vi "Create Tones.vi"(0 "ToneCloud in":refnum<class "Tone Cloud.lvclass">, 9 "Fs (Hz)":dbl, 11 "error in (no error)":errorcluster) -> (4 "ToneCloud out":refnum<class "Tone Cloud.lvclass">, 15 "error out":errorcluster)   [LabVIEW 2020, in "Tone Cloud.lvclass"]
uses:
  Tone Cloud.lvclass
  Tone Cloud.lvclass/Tone Cloud.ctl
  <vilib>/Analysis/NI_AALBase.lvlib
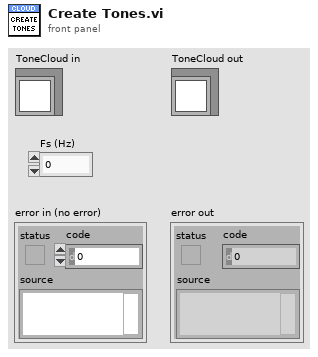
[diagram p1: front panel]
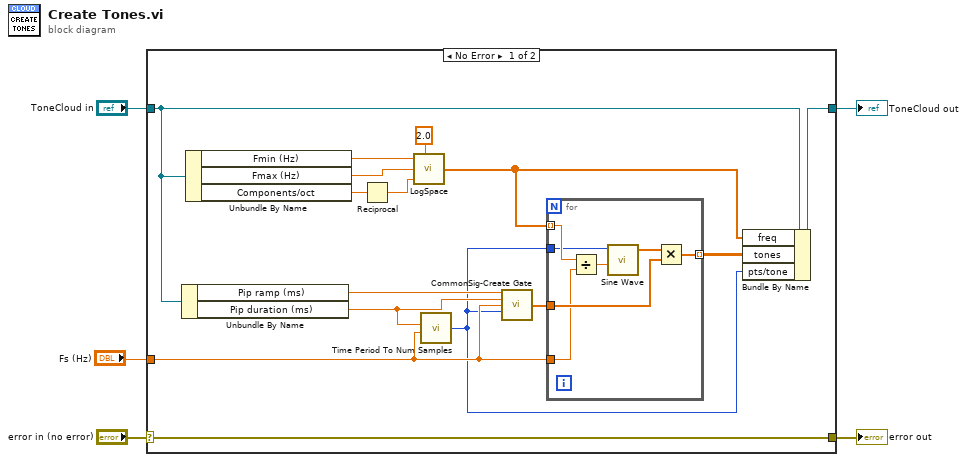
[diagram p0: block diagram]
diagram:
  n1 = case shown="No Error" "error in (no error)" {
    selector: "error in (no error)" -> [w20 w29]
    tunnel: [w20 w29] -> w4
    tunnel: [w10 w28] -> w2
    tunnel: "ToneCloud in" -> [w9 w28]
    tunnel: "Fs (Hz)" -> [w8 _]
    frame No Error {
      n2 = Unbundle By Name(w9) -> ("Pip ramp (ms)"=w11:dbl, "Pip duration (ms)"=w14:dbl)
      n3 = Unbundle By Name(w9) -> ("Fmin (Hz)"=w17:dbl, "Fmax (Hz)"=w18:dbl, "Components/oct"=w19:dbl)
      n4 = Reciprocal(x=w19) -> (1/x=w16:dbl)
      n5 = call "LogSpace.vi"("Start"=w17, "Base"=2.0, "Stop"=w18, "Step"=w16) -> ("Array"=w6:dbl[])  [unwired: 2 in, 1 out]
      n6 = call "Time Period To Num Samples.vi"("Duration (ms)"=w14, "Sampling rate (Hz)"=w8) -> ("Samples"=w7:i32)  [unwired: 5 in]
      n7 = call "CommonSig-Create Gate.vi"("Ramp (ms)"=w11, "Duration (ms)"=w14, "Sampling Rate (Hz)"=w8, "Npts"=w7) -> ("Gate"=w12:dbl[])  [unwired: 10 in, 1 out]
      n8 = for {
        tunnel: w6 -> [w25] mode=indexing
        tunnel: w12 -> [w27]
        tunnel: w7 -> [w22]
        tunnel: [w26] -> w13 mode=indexing
        tunnel: w8 -> [w24]
        n9 = Divide(x=w25, y=w24) -> (x/y=w23:dbl)
        n10 = call <vilib>:"Sine Wave.vi"("samples"=w22, "frequency"=w23) -> ("sine wave"=w21:dbl[])  [unwired: 3 in, 2 out]
        n11 = Multiply(x=w21, y=w27) -> (x*y=w26:dbl[])
      }
      n12 = Bundle By Name(cluster=w9, "freq"=w6, "tones"=w13, "pts/tone"=w7) -> (w10:refnum<class "Tone Cloud.lvclass">)
    }
    frame Error {
    }
  }
  "error out" <- w4
  "ToneCloud out" <- w2
